vi "LC1_MS_Main.vi"(0 "MS_Network_Settings":T5, 1 "Analog Output":T1[](array[typedef]) {"value" format="%#_15f"}, 2 "Analog Input Indexes":u16[](array[numeric]), 3 "Digital Input Indexes":u16[](array[numeric]), 5 "MS_DNP3_Settings":T15={"Binary Out Mode"=6, "Binary In Variation"=0, "Analog Out Variation"=4, "Analog Out Mode"=6, "Analog In Variation"=6} {"Binary Out Mode" items=["SBO"=0, "Select"=3, "Operate"=4, "Direct"=5, "Direct No Ack"=6]; "Binary In Variation" items=["Default", "Packed Format", "With Flags"]; "Analog Out Variation" items=["32-bit"=1, "16-bit"=2, "Single-prec"=3, "Double-prec"=4]; "Analog Out Mode" items=["SBO"=0, "Select"=3, "Operate"=4, "Direct"=5, "Direct No Ack"=6]; "Analog In Variation" items=["Default", "32-bit with Flag", "16-bit with Flag", "32-bit without Flag", "16-bit without Flag", "Single-prec with Flag", "Double-prec with Flag"]}, 7 "MS_RESET":bool, 9 "MS_ENABLE":bool, 11 "Poll Enable":T13, 13 "Digital Output":T6[](array[typedef]) {"CROB value"."Control" items=["Nul"=0, "Pulse On"=1, "Pulse Off"=2, "Latch On"=3, "Latch Off"=4, "Close"=65, "Trip"=129]}, 14 "DNP3 Session Feedback":T4) -> (4 "Comm Status":T14, 6 "Analog Input":dbl[](array[numeric]), 8 "Digital Input":bool[](array[boolean]), 15 "DNP3 Session Output":T4)   [LabVIEW 2016, in "DNP3_Master_Station_MGCC.lvlib"]
uses:
  DNP3_Master_Station_MGCC.lvlib
  Tab_Master.ctl
  <vilib>/DNP3/DNP3_Master/Operation Mode.ctl
  <vilib>/DNP3/DNP3_Master/Poll Binary Input Variation.ctl
  <vilib>/DNP3/DNP3_Master/Analog Variation.ctl
  <vilib>/DNP3/DNP3_Master/Poll Analog Input Variation.ctl
  <vilib>/DNP3/DNP3_Master/Response Type.ctl
  <vilib>/DNP3/DNP3_Master/Analog Info.ctl
  <vilib>/DNP3/DNP3_Master/Start Stop.ctl
  <vilib>/DNP3/DNP3_Master/Crob With Index.ctl
  <vilib>/DNP3/DNP3_Common/crob.ctl
  <vilib>/DNP3/DNP3_Common/crob_ctrl.ctl
  <vilib>/Utility/error.llb/Error Cluster From Error Code.vi
  <vilib>/DNP3/DNP3_Master/Send CROB (Blocking).vi
  <vilib>/DNP3/DNP3_Master/Read Binary Input.vi
  <vilib>/DNP3/DNP3_Master/Send Poll Binary Input By StartStop (Blocking).vi
  <vilib>/DNP3/DNP3_Master/Send Analog Output Block (Blocking).vi
  <vilib>/DNP3/DNP3_Master/Read Analog Input.vi
  <vilib>/DNP3/DNP3_Master/Send Poll Analog Input By StartStop (Blocking).vi
  <vilib>/DNP3/DNP3_Master/Send Poll Analog Input By AllPoints (Blocking).vi
  <vilib>/ErrorRing/Error Ring.xnode
  <vilib>/DNP3/DNP3_Master.lvlib
  <resource>/objmgr/dnp3.rc
  <vilib>/DNP3/DNP3_Common.lvlib
panel:
  out "array w/ subset deleted":T1[](array[typedef]) {"value" format="%#_15f"}
  out "MS_Network_Settings_Initial 3":T5
  out "MS_Network_Settings_Initial 2":T5
  out "Ping status":T2=enum."Cancel"
  out "PollD":T3[](array[typedef])
  out "Array":T3[](array[typedef])
  out "PollA":T3[](array[typedef])
  out "Binary Out Mode":T9=6 items=["SBO"=0, "Select"=3, "Operate"=4, "Direct"=5, "Direct No Ack"=6]
  out "Binary In Variation":T10 items=["Default", "Packed Format", "With Flags"]
  out "Analog Out Variation":T11=4 items=["32-bit"=1, "16-bit"=2, "Single-prec"=3, "Double-prec"=4]
  out "Analog Out Mode":T9 items=["SBO"=0, "Select"=3, "Operate"=4, "Direct"=5, "Direct No Ack"=6]
  out "Analog In Variation":T12 items=["Default", "32-bit with Flag", "16-bit with Flag", "32-bit without Flag", "16-bit without Flag", "Single-prec with Flag", "Double-prec with Flag"]
  out "MS_TX_Status_Binary":T2
  out "MS_TX_Status_Analog":T2
  out "MS_RX_Status_Binary":T2
  out "MS_RX_Status_Analog":T2
  out "MS_Network_Settings_Initial":T5
  in  "En_Tx_Di":bool
  in  "En_Tx_An":bool
  in  "En_Rx_Di":bool
  in  "En_Rx_An":bool
  out "MS_RESET_IND":bool
  out "object flags":u8[](array[numeric]) format="%08b"
  in  "Channel Setting":T16
  in  "serial port":u16=1
  in  "baud rate (9600)":u32=9600
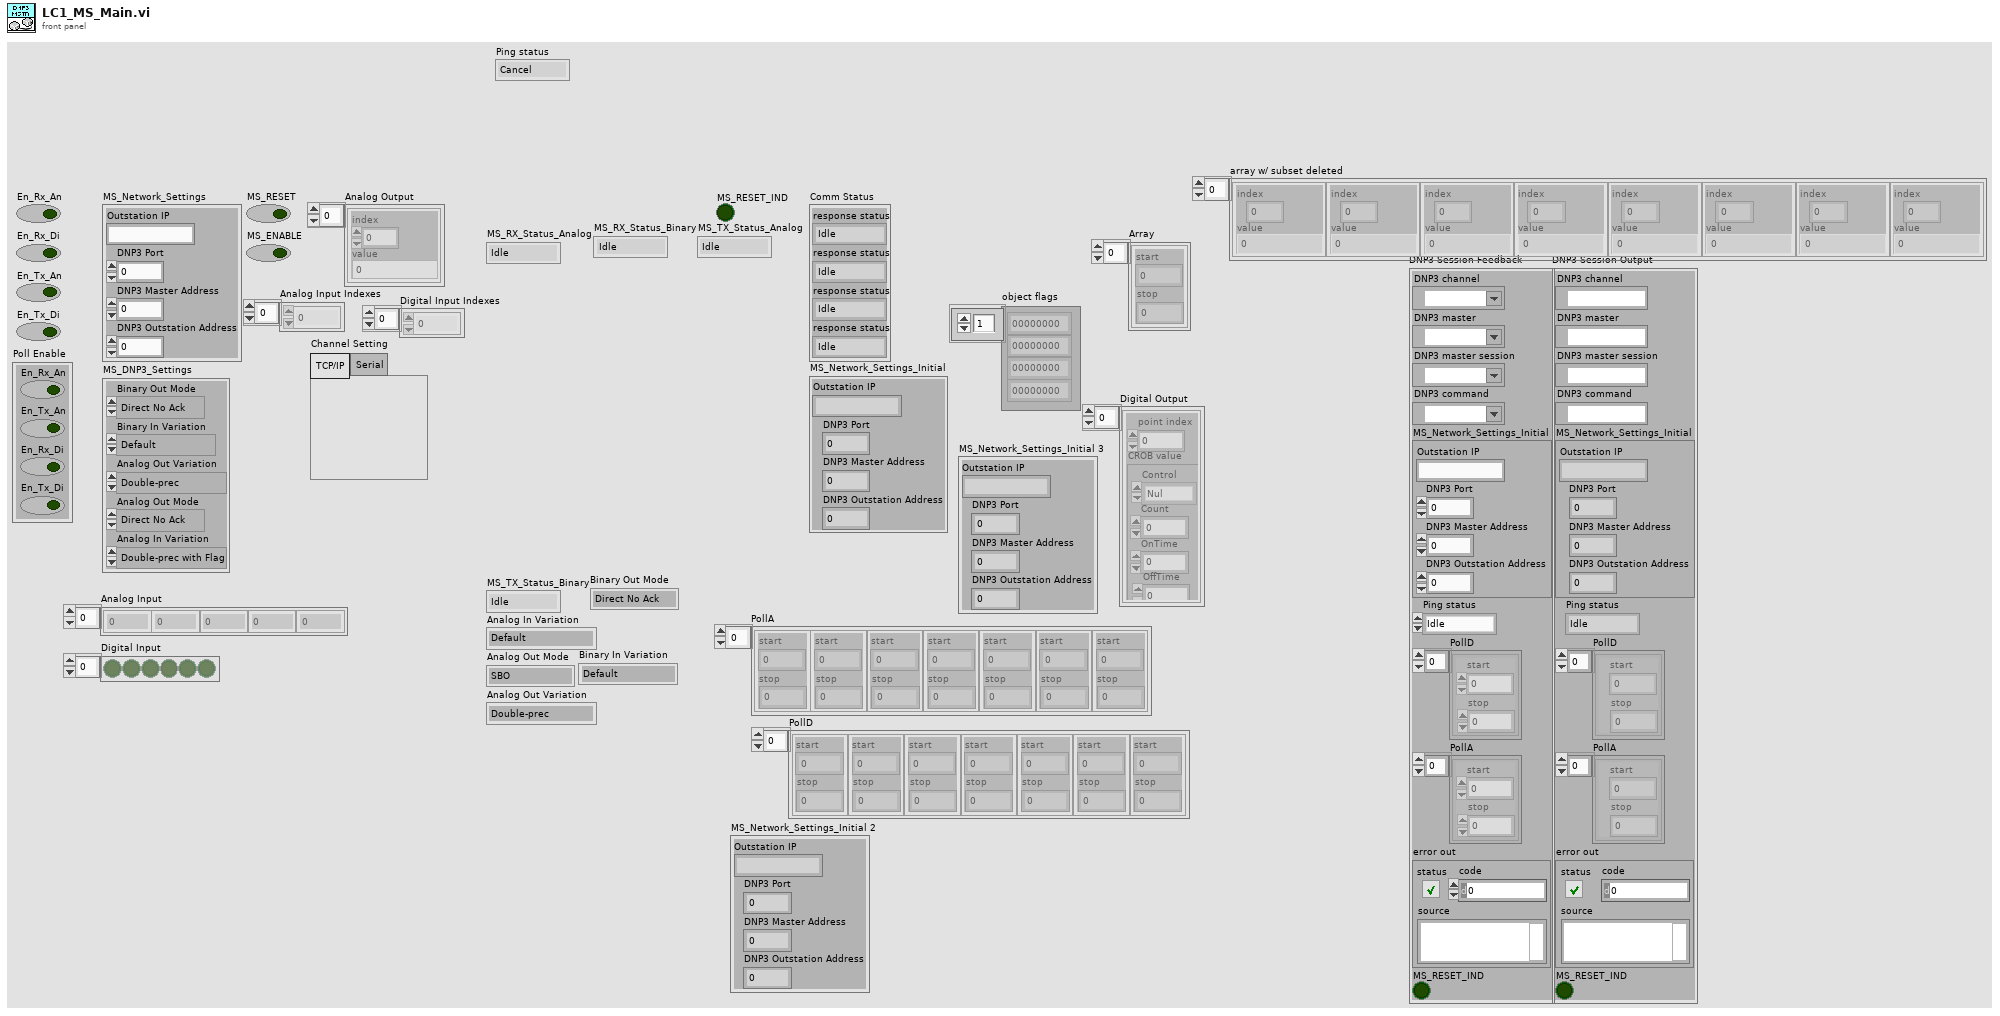
[diagram p1: front panel]
types:
  T1 = typedef "DNP3_Master.lvlib/Analog Info.ctl" = cluster{"index":u16, "value":dbl}
  T2 = typedef "DNP3_Master.lvlib/Response Type.ctl" = enum16{"Idle", "Buffering", "Pending", "Success", "Failure", "Mismatch", "Status Code", "IIN", "Timeout", "Cancel"}
  T3 = typedef "DNP3_Master.lvlib/Start Stop.ctl" = cluster{"start":u16, "stop":u16}
  T4 = cluster{"DNP3 channel":refnum<k21>, "DNP3 master":refnum<k21>, "DNP3 master session":refnum<k21>, "DNP3 command":refnum<k21>, "MS_Network_Settings_Initial":cluster{"Outstation IP":string, "DNP3 Port":u16, "DNP3 Master Address":u16, "DNP3 Outstation Address":u16}, "Ping status":T2, "PollD":T3[], "PollA":T3[], "error out":errorcluster, "MS_RESET_IND":bool}
  T5 = cluster{"Outstation IP":string, "DNP3 Port":u16, "DNP3 Master Address":u16, "DNP3 Outstation Address":u16}
  T6 = typedef "DNP3_Master.lvlib/Crob With Index.ctl" = cluster{"point index":u16, "CROB value":T7}
  T7 = typedef "DNP3_Common.lvlib/crob.ctl" = cluster{"OnTime":u32, "Count":u8, "OffTime":u32, "Control":T8}
  T8 = typedef "DNP3_Common.lvlib/crob_ctrl.ctl" = u8
  T9 = typedef "DNP3_Master.lvlib/Operation Mode.ctl" = u8
  T10 = typedef "DNP3_Master.lvlib/Poll Binary Input Variation.ctl" = u8
  T11 = typedef "DNP3_Master.lvlib/Analog Variation.ctl" = u8
  T12 = typedef "DNP3_Master.lvlib/Poll Analog Input Variation.ctl" = u8
  T13 = cluster{"En_Rx_An":bool, "En_Tx_An":bool, "En_Rx_Di":bool, "En_Tx_Di":bool}
  T14 = cluster{"response status":T2, "response status":T2, "response status":T2, "response status":T2}
  T15 = cluster{"Binary Out Mode":T9, "Binary In Variation":T10, "Analog Out Variation":T11, "Analog Out Mode":T9, "Analog In Variation":T12}
  T16 = typedef "Tab_Master.ctl" = enum32{"TCP/IP", "Serial"}
  T17 = cluster{"Analog RX":T2, "Analog RX":T2, "Analog RX":T2, "Analog RX":T2}
  T18 = cluster{"DNP3 Master Address":u16, "DNP3 Outstation Address":u16}
  T19 = cluster{"x = y?":bool, "Outstation IP":string, "DNP3 Port":u16, "serial port":u16, "baud rate (9600)":u32}
  T20 = cluster{"MS_RX_Status_Analog":T2, "MS_TX_Status_Analog":T2, "MS_RX_Status_Binary":T2, "MS_TX_Status_Binary":T2}
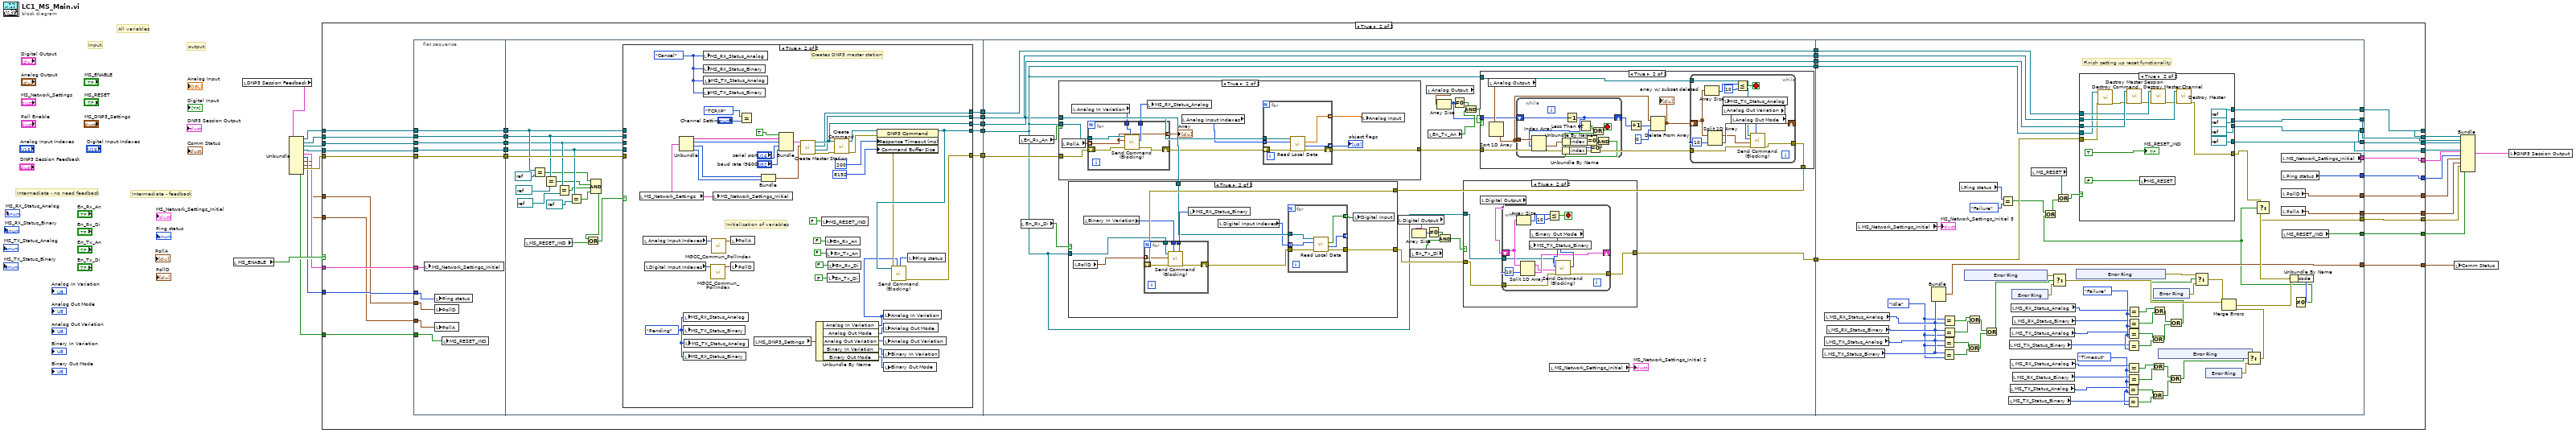
[diagram p0: block diagram]
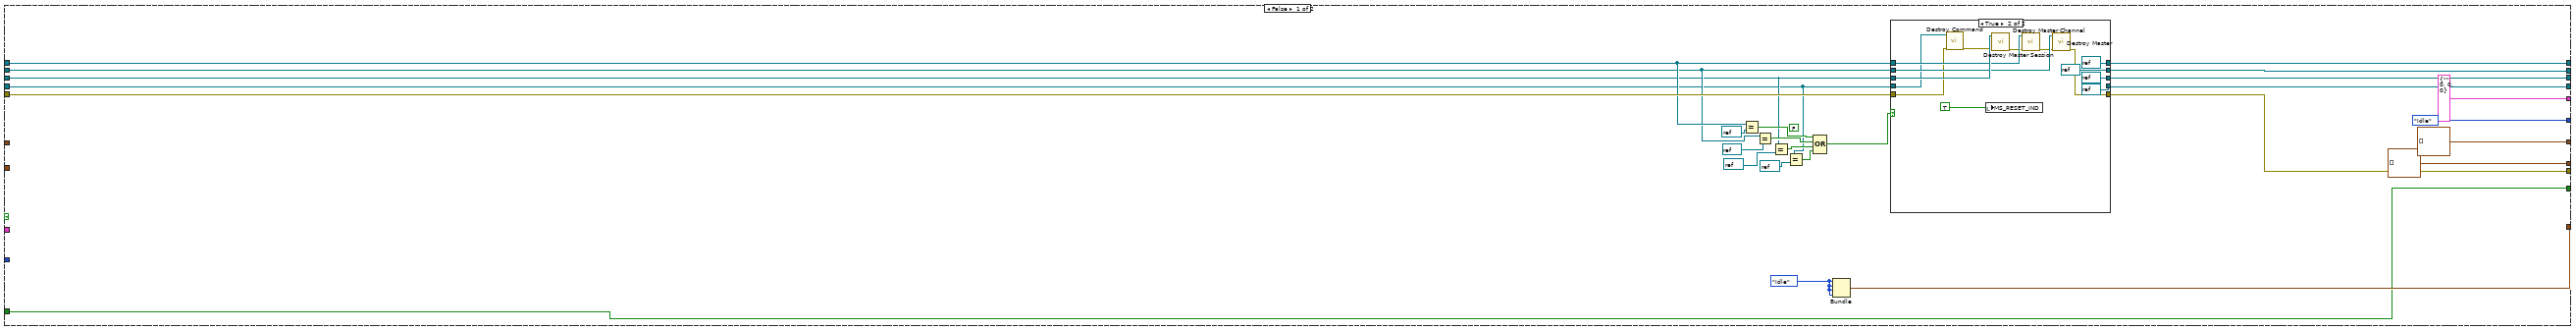
[diagram p2: hidden frame]
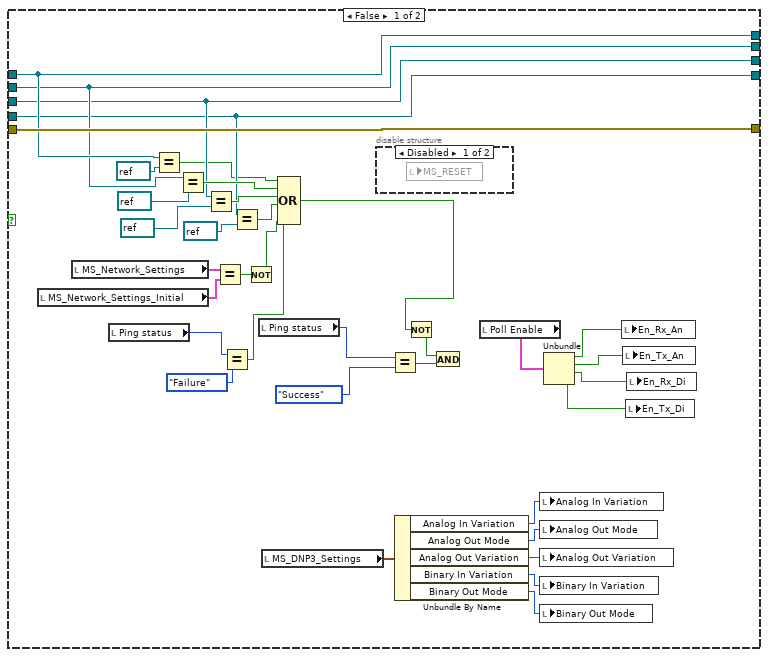
[diagram p4: hidden frame]
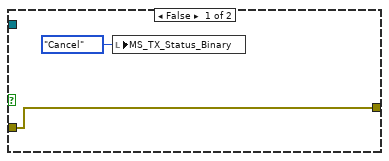
[diagram p6: hidden frame]
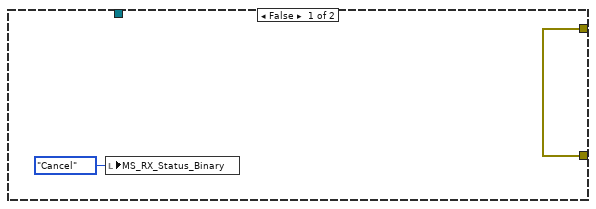
[diagram p7: hidden frame]
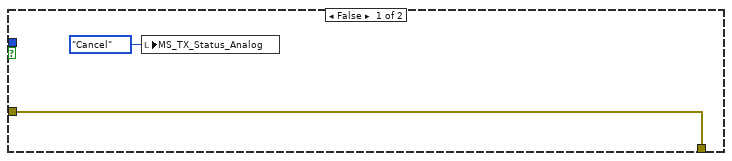
[diagram p8: hidden frame]
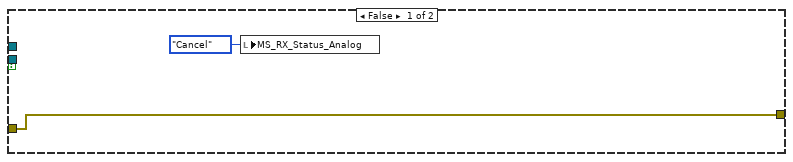
[diagram p9: hidden frame]
diagram:
  # "Intermediate - feedback"
  # "Intermediate - no need feedback"
  # "output"
  # "Input"
  # "All variables"
  n1 = local read "MS_ENABLE"() -> (w17:bool)
  n2 = local read "DNP3 Session Feedback"() -> (w9:T4)
  n3 = Unbundle(w9) -> ("DNP3 channel"=w24:refnum<k21>, "DNP3 master"=w23:refnum<k21>, "DNP3 master session"=w21:refnum<k21>, "DNP3 command"=w22:refnum<k21>, "MS_Network_Settings_Initial"=w7:T5, "Ping status"=w6:T2, "PollD"=w5:T3[], "PollA"=w4:T3[], "error out"=w8:errorcluster, "MS_RESET_IND"=w1:bool)
  n4 = case shown="True" w17 {
    tunnel: w23 -> [w32 w105]
    tunnel: w21 -> [w31 w104]
    tunnel: w22 -> [w30 w103]
    tunnel: [w45 w86] -> w19
    tunnel: w8 -> [w48 w102]
    tunnel: [w47 w89] -> w10
    tunnel: [w44 w85] -> w18
    tunnel: [w43 w88] -> w15
    tunnel: [w46 w87] -> w20
    tunnel: w24 -> [w33 w101]
    tunnel: [w50 w90] -> w16
    tunnel: [T5 {"Outstation IP"="", "DNP3 Port"=0, "DNP3 Master Address"=0, "DNP3 Outstation Address"=0} ("MS_Network_Settings_Initial") w75] -> w14
    tunnel: [Response_Type."Idle" ("Ping status") w74] -> w13
    tunnel: [T3[] [] ("PollD") w73] -> w12
    tunnel: [T3[] [] ("PollA") w72] -> w11
    tunnel: w7 -> [_ w84]
    tunnel: w6 -> [_ w83]
    tunnel: w5 -> [_ w82]
    tunnel: w4 -> [_ w81]
    tunnel: [w25 w71] -> w3
    tunnel: w1 -> [w25 w70]
    frame False {
      (unwired) FALSE ("value")
      w49 = Response_Type."Idle" ("Analog RX")
      n5 = Equal?(x=w33, y=refnum<k21> refnum ("DNP3 channel")) -> (x = y?=w35:bool)
      n6 = Equal?(x=w32, y=refnum<k21> refnum) -> (x = y?=w37:bool)
      n7 = Equal?(x=w31, y=refnum<k21> refnum) -> (x = y?=w38:bool)
      n8 = Equal?(x=w30, y=refnum<k21> refnum) -> (x = y?=w39:bool)
      n9 = Compound Arithmetic op=OR(w35, w37, w38, w39) -> (w34:bool)
      n10 = Bundle("Analog RX"=w49, "Analog RX"=w49, "Analog RX"=w49, "Analog RX"=w49) -> (w50:T17)  [unwired: 1 in]
      n11 = case shown="True" w34 {
        tunnel: w31 -> [w52 w69]
        tunnel: w48 -> [w55 w61]
        tunnel: w33 -> [w54 w68]
        tunnel: w32 -> [w53 w67]
        tunnel: [w55 w66] -> w47
        tunnel: w30 -> [w51 w62]
        tunnel: [w54 refnum<k21> refnum ("DNP3 channel")] -> w46
        tunnel: [w53 refnum<k21> refnum ("DNP3 master")] -> w45
        tunnel: [w52 refnum<k21> refnum ("DNP3 master session")] -> w44
        tunnel: [w51 refnum<k21> refnum ("DNP3 command")] -> w43
        frame False {
        }
        frame True {
          n12 = call <vilib>:"Destroy Command.vi"("error in (no error)"=w61, "DNP3 command in"=w62) -> ("error out"=w60:errorcluster)  [unwired: 8 in, 1 out]
          n13 = local write "MS_RESET_IND"(TRUE ("MS_Comm_Reset_Succesful")) -> ()
          n14 = call <vilib>:"Destroy Master Session.vi"("error in (no error)"=w60, "DNP3 master session in"=w69) -> ("error out"=w65:errorcluster)  [unwired: 8 in, 1 out]
          n15 = call <vilib>:"Destroy Master Channel.vi"("error in (no error)"=w65, "DNP3 channel in"=w68) -> ("error out"=w64:errorcluster)  [unwired: 8 in, 1 out]
          n16 = call <vilib>:"Destroy Master.vi"("error in (no error)"=w64, "DNP3 master"=w67) -> ("error out"=w66:errorcluster)  [unwired: 9 in]
        }
      }
    }
    frame True {
      n17 = flat-sequence {
        tunnel: w81 -> [w107]
        tunnel: w82 -> [w108]
        tunnel: w83 -> [w109]
        tunnel: w84 -> [w110]
        tunnel: w101 -> [w111]
        tunnel: w102 -> [w112]
        tunnel: w103 -> [w113]
        tunnel: w104 -> [w114]
        tunnel: w105 -> [w115]
        tunnel: [w115] -> w80
        tunnel: [w114] -> w79
        tunnel: [w113] -> w78
        tunnel: [w112] -> w77
        tunnel: [w111] -> w76
        tunnel: w70 -> [w106]
        tunnel: [w136] -> w100
        tunnel: [w135] -> w99
        tunnel: [w133] -> w98
        tunnel: [w132] -> w97
        tunnel: [w131] -> w96
        tunnel: w80 -> [w126]
        tunnel: w79 -> [w125]
        tunnel: w78 -> [w124]
        tunnel: w77 -> [w134]
        tunnel: w76 -> [w129]
        tunnel: w100 -> [w221]
        tunnel: w99 -> [w219]
        tunnel: w98 -> [w217]
        tunnel: w97 -> [w220]
        tunnel: w96 -> [w218]
        tunnel: [w220] -> w95
        tunnel: [w219] -> w94
        tunnel: [w218] -> w93
        tunnel: [w217] -> w92
        tunnel: [w216] -> w91
        tunnel: w95 -> [w411]
        tunnel: w94 -> [w410]
        tunnel: w93 -> [w409]
        tunnel: w92 -> [w408]
        tunnel: w91 -> [w407]
        tunnel: [w360] -> w90
        tunnel: [w359] -> w89
        tunnel: [w358] -> w88
        tunnel: [w356] -> w87
        tunnel: [w355] -> w86
        tunnel: [w354] -> w85
        tunnel: [w351] -> w75
        tunnel: [w350] -> w74
        tunnel: [w349] -> w73
        tunnel: [w348] -> w72
        tunnel: [w347] -> w71
        frame #0 {
          n18 = local write "MS_Network_Settings_Initial"(w110) -> ()
          n19 = local write "Ping status"(w109) -> ()
          n20 = local write "PollD"(w108) -> ()
          n21 = local write "PollA"(w107) -> ()
          n22 = local write "MS_RESET_IND"(w106) -> ()
        }
        frame #1 {
          n23 = local read "MS_RESET_IND"() -> (w130:bool)
          n24 = Equal?(x=w129, y=refnum<k21> refnum ("DNP3 channel")) -> (x = y?=w123:bool)
          n25 = Equal?(x=w126, y=refnum<k21> refnum) -> (x = y?=w122:bool)
          n26 = Equal?(x=w125, y=refnum<k21> refnum) -> (x = y?=w121:bool)
          n27 = Equal?(x=w124, y=refnum<k21> refnum) -> (x = y?=w120:bool)
          n28 = Compound Arithmetic op=AND(w123, w122, w121, w120) -> (w116:bool)
          n29 = Or(x=w116, y=w130) -> (x .or. y?=w127:bool)
          n30 = case shown="True" w127 {
            tunnel: [w172 w192] -> w136
            tunnel: [w153 w194] -> w131
            tunnel: [w154 w208] -> w133
            tunnel: w126 -> [w155 _]
            tunnel: w125 -> [w154 _]
            tunnel: w124 -> [w153 _]
            tunnel: [w155 w195] -> w135
            tunnel: w134 -> [w172 _]
            tunnel: [w156 w196] -> w132
            tunnel: w129 -> [w156 _]
            frame False {
              n31 = local read "MS_Network_Settings_Initial"() -> (w147:T5)
              n32 = local read "MS_Network_Settings"() -> (w148:T5)
              n33 = local read "Ping status"() -> (w144:T2)
              n34 = Equal?(x=w156, y=refnum<k21> refnum ("DNP3 channel")) -> (x = y?=w152:bool)
              n35 = Equal?(x=w155, y=refnum<k21> refnum) -> (x = y?=w158:bool)
              n36 = Equal?(x=w154, y=refnum<k21> refnum) -> (x = y?=w159:bool)
              n37 = Equal?(x=w148, y=w147) -> (x = y?=w149:bool)
              n38 = Equal?(x=w144, y=Response_Type."Failure" ("Ping status")) -> (x = y?=w142:bool)
              n39 = Equal?(x=w153, y=refnum<k21> refnum) -> (x = y?=w160:bool)
              n40 = Not(x=w149) -> (.not. x?=w146:bool)
              n41 = local read "Ping status"() -> (w171:T2)
              n42 = local read "MS_DNP3_Settings"() -> (w169:T15)
              n43 = Compound Arithmetic op=OR(w152, w158, w159, w160, w146, w142) -> (w145:bool)
              n44 = disable-structure shown="Disabled" {
                frame Disabled {
                  n45 = local read "MS_RESET"() -> ()  [unwired: 1 in]
                }
                frame Enabled {
                }
              }
              n46 = Equal?(x=w171, y=Response_Type."Success" ("Ping status")) -> (x = y?=w151:bool)
              n47 = Unbundle By Name(w169) -> ("Analog In Variation"=w168:T12, "Analog Out Mode"=w167:T9, "Analog Out Variation"=w166:T11, "Binary In Variation"=w165:T10, "Binary Out Mode"=w164:T9)
              n48 = Not(x=w145) -> (.not. x?=w150:bool)
              n49 = And(x=w150, y=w151) -> ()  [unwired: 1 out]
              n50 = local read "Poll Enable"() -> (w137:T13)
              n51 = local write "Analog In Variation"(w168) -> ()
              n52 = local write "Analog Out Mode"(w167) -> ()
              n53 = local write "Analog Out Variation"(w166) -> ()
              n54 = local write "Binary In Variation"(w165) -> ()
              n55 = local write "Binary Out Mode"(w164) -> ()
              n56 = Unbundle(w137) -> ("En_Rx_An"=w138:bool, "En_Tx_An"=w139:bool, "En_Rx_Di"=w140:bool, "En_Tx_Di"=w141:bool)
              n57 = local write "En_Rx_An"(w138) -> ()
              n58 = local write "En_Tx_An"(w139) -> ()
              n59 = local write "En_Tx_Di"(w141) -> ()
              n60 = local write "En_Rx_Di"(w140) -> ()
            }
            frame True {
              w182 = Response_Type."Pending" ("LC1_MS_RX_Status_Binary")
              w197 = Response_Type."Cancel" ("LC1_MS_RX_Status_Binary")
              # "Initialization of variables"
              # "Creates DNP3 master station"
              n61 = local read "MS_Network_Settings"() -> (w180:T5)
              n62 = local read "Analog Input Indexes"() -> (w187:u16[])
              n63 = local read "Digital Input Indexes"() -> (w186:u16[])
              n64 = Unbundle(w180) -> ("Outstation IP"=w207:string, "DNP3 Port"=w206:u16, "DNP3 Master Address"=w205:u16, "DNP3 Outstation Address"=w204:u16)
              n65 = local write "MS_RX_Status_Analog"(w182) -> ()
              n66 = local write "MS_TX_Status_Binary"(w182) -> ()
              n67 = local write "MS_RX_Status_Binary"(w182) -> ()
              n68 = local write "MS_TX_Status_Analog"(w182) -> ()
              n69 = local write "MS_RX_Status_Analog"(w197) -> ()
              n70 = local write "MS_RX_Status_Binary"(w197) -> ()
              n71 = local write "MS_TX_Status_Binary"(w197) -> ()
              n72 = local write "MS_TX_Status_Analog"(w197) -> ()
              n73 = call "MGCC_Commun_PollIndex.vi"("Analog Input Indexes"=w186) -> ("Poll"=w183:T3[])  [unwired: 10 in]
              n74 = call "MGCC_Commun_PollIndex.vi"("Analog Input Indexes"=w187) -> ("Poll"=w184:T3[])  [unwired: 10 in]
              n75 = local write "MS_Network_Settings_Initial"(w180) -> ()
              n76 = local write "PollD"(w183) -> ()
              n77 = local write "PollA"(w184) -> ()
              n78 = Equal?(x=Tab_Master."TCP/IP" ("Channel Setting"), y="Channel Setting") -> ()  [unwired: 1 out]
              n79 = local read "MS_DNP3_Settings"() -> (w179:T15)
              n80 = Bundle("DNP3 Master Address"=w205, "DNP3 Outstation Address"=w204) -> (w202:T18)  [unwired: 1 in]
              n81 = Bundle("x = y?"=TRUE, "Outstation IP"=w207, "DNP3 Port"=w206, "serial port"="serial port", "baud rate (9600)"="baud rate (9600)") -> (w203:T19)  [unwired: 1 in]
              n82 = call "Create Master Station.vi"("Session Cluster"=w202, "Channel Cluster"=w203) -> ("error out"=w210:errorcluster, "DNP3 master"=w195:refnum<k21>, "DNP3 channel"=w196:refnum<k21>, "DNP3 master session"=w208:refnum<k21>)  [unwired: 3 in]
              n83 = Unbundle By Name(w179) -> ("Analog In Variation"=w174:T12, "Analog Out Mode"=w178:T9, "Analog Out Variation"=w177:T11, "Binary In Variation"=w176:T10, "Binary Out Mode"=w175:T9)
              n84 = local write "MS_RESET_IND"(FALSE ("MS_Comm_Reset_Ind")) -> ()
              n85 = local write "En_Rx_An"(FALSE ("En_Rx_An")) -> ()
              n86 = local write "En_Tx_An"(FALSE ("En_Tx_An")) -> ()
              n87 = local write "En_Tx_Di"(FALSE ("En_Tx_Di")) -> ()
              n88 = local write "En_Rx_Di"(FALSE ("En_Rx_Di")) -> ()
              n89 = call <vilib>:"Create Command.vi"("error in (no error)"=w210, "DNP3 master session"=w208) -> ("error out"=w200:errorcluster, "DNP3 command"=w201:refnum<k21>)  [unwired: 8 in]
              n90 = property class="DNP3 Command"(reference=w201, error in=w200, "Response Timeout (ms)"=u32 200 ("Misc:Response Timeout (ms)"), "Command Buffer Size"=u32 8192 ("Misc:Command Buffer Size")) -> (reference out=w194:refnum<k21>, error out=w193:errorcluster)
              n91 = local write "Analog In Variation"(w174) -> ()
              n92 = local write "Analog Out Mode"(w178) -> ()
              n93 = local write "Analog Out Variation"(w177) -> ()
              n94 = local write "Binary In Variation"(w176) -> ()
              n95 = local write "Binary Out Mode"(w175) -> ()
              n96 = call-poly <vilib>:"Send Command (Blocking).vi"("variation (Default)"=w174, "error in (no error)"=w193, "DNP3 command in"=w194) -> ("error out"=w192:errorcluster, "response status"=w181:T2)  [unwired: 6 in, 1 out]
              n97 = local write "Ping status"(w181) -> ()
            }
          }
        }
        frame #2 {
          n98 = local read "En_Rx_An"() -> (w232:bool)
          n99 = local read "En_Rx_Di"() -> (w233:bool)
          n100 = case shown="True" w232 {
            tunnel: w221 -> [w316 w328]
            tunnel: w217 -> [_ w322]
            tunnel: w218 -> [_ w327]
            tunnel: [w316 w325] -> w222
            frame False {
              n101 = local write "MS_RX_Status_Analog"(Response_Type."Cancel" ("MS_RX_Status_Analog")) -> ()
            }
            frame True {
              n102 = local read "PollA"() -> (w320:T3[])
              n103 = local read "Analog In Variation"() -> (w323:T12)
              n104 = for {
                tunnel: w327 -> [w333]
                tunnel: [w332] -> w324
                tunnel: w323 -> [w331]
                shift-right: [w330] -> w321
                shift-left: w328 -> [w334]
                tunnel: w320 -> [w329] mode=indexing
                tunnel: [w329] -> w318 mode=indexing
                n105 = call-poly <vilib>:"Send Command (Blocking).vi"("variation (Default)"=w331, "error in (no error)"=w334, "range"=w329, "DNP3 command in"=w333) -> ("error out"=w330:errorcluster, "response status"=w332:T2)  [unwired: 5 in, 1 out]
              }
              "Array" <- w318
              n106 = local write "MS_RX_Status_Analog"(w324) -> ()
              n107 = local read "Analog Input Indexes"() -> (w319:u16[])
              n108 = for {
                tunnel: [w338] -> w317 mode=indexing
                tunnel: [w337] -> w326 mode=indexing
                tunnel: w322 -> [w336]
                tunnel: w319 -> [w335] mode=indexing
                shift-right: [w339] -> w325
                shift-left: w321 -> [w340]
                n109 = call-poly <vilib>:"Read Local Data.vi"("error in (no error)"=w340, "point index"=w335, "DNP3 master session in"=w336) -> ("error out"=w339:errorcluster, "object flags"=w337:u8, "value"=w338:dbl)  [unwired: 5 in, 1 out]
              }
              "object flags" <- w326
              n110 = local write "Analog Input"(w317) -> ()
            }
          }
          n111 = local read "Digital Output"() -> (w231:T6[])
          n112 = local read "En_Tx_Di"() -> (w235:bool)
          n113 = Array Size(array=w231) -> (size(s)=w228:i32)
          n114 = local read "Analog Output"() -> (w227:T1[])
          n115 = Not Equal To 0?(x=w228) -> (x != 0?=w229:bool)
          n116 = local read "En_Tx_An"() -> (w234:bool)
          n117 = Array Size(array=w227) -> (size(s)=w214:i32)
          n118 = And(x=w229, y=w235) -> (x .and. y?=w230:bool)
          n119 = Not Equal To 0?(x=w214) -> (x != 0?=w226:bool)
          n120 = And(x=w226, y=w234) -> (x .and. y?=w225:bool)
          n121 = case shown="True" w225 {
            tunnel: w218 -> [_ w288]
            tunnel: w222 -> [w279 w289]
            tunnel: [w279 w287] -> w223
            tunnel: w214 -> [_ w283]
            frame False {
              n122 = local write "MS_TX_Status_Analog"(Response_Type."Cancel" ("MS_TX_Status_Analog")) -> ()
            }
            frame True {
              n123 = local read "Analog Output"() -> (w284:T1[])
              n124 = Sort 1D Array(array=w284) -> (sorted array=w280:T1[])
              n125 = while {
                shift-right: [w290] -> w281
                shift-left: w283 -> [w297]
                tunnel: w280 -> [w295]
                stop <- w301 stop-if-true
                n126 = Decrement(x=w297) -> (x-1=w290:i32)
                n127 = Index Array(array=w295, index #1=w290) -> (element #1=w292:T1, element #2=w291:T1)  [unwired: 1 in]
                n128 = Unbundle By Name(w291) -> ("index"=w294:u16)
                n129 = Unbundle By Name(w292) -> ("index"=w293:u16)
                n130 = Less Than 0?(x=w290) -> (x < 0?=w296:bool)
                n131 = Equal To 0?(x=w293) -> (x = 0?=w300:bool)
                n132 = Equal To 0?(x=w294) -> (x = 0?=w299:bool)
                n133 = And(x=w300, y=w299) -> (x .and. y?=w298:bool)
                n134 = Or(x=w296, y=w298) -> (x .or. y?=w301:bool)
              }
              n135 = Increment(x=w281) -> (x+1=w282:i32)
              n136 = Delete From Array(array=w280, length=w282, index=0) -> (array with subset deleted=w286:T1[])  [unwired: 1 out]
              "array w/ subset deleted" <- w286
              n137 = while {
                shift-right: [w306] -> _
                shift-left: w286 -> [w310]
                tunnel: [w305] -> w287
                tunnel: w288 -> [w304]
                tunnel: w289 -> [w302]
                stop <- w311 stop-if-true
                n138 = Array Size(array=w310) -> (size(s)=w313:i32)
                n139 = Split 1D Array(array=w310, index=10) -> (first subarray=w303:T1[], second subarray=w306:T1[])
                n140 = local read "Analog Out Variation"() -> (w307:T11)
                n141 = local read "Analog Out Mode"() -> (w308:T9)
                n142 = Less Or Equal?(x=w313, y=10) -> (x <= y?=w311:bool)
                n143 = call-poly <vilib>:"Send Command (Blocking).vi"("variation"=w307, "error in (no error)"=w302, "values"=w303, "mode"=w308, "DNP3 command in"=w304) -> ("error out"=w305:errorcluster, "response status"=w309:T2)  [unwired: 4 in, 1 out]
                n144 = local write "MS_TX_Status_Analog"(w309) -> ()
              }
            }
          }
          n145 = case shown="True" w233 {
            tunnel: w217 -> [_ w260]
            tunnel: w218 -> [_ w257]
            tunnel: w223 -> [w255 w265]
            tunnel: [w255 w264] -> w224
            frame False {
              n146 = local write "MS_RX_Status_Binary"(Response_Type."Cancel" ("MS_RX_Status_Binary")) -> ()
            }
            frame True {
              n147 = local read "PollD"() -> (w258:T3[])
              n148 = local read "Binary In Variation"() -> (w261:T10)
              n149 = for {
                tunnel: [w269] -> w262
                tunnel: w261 -> [w268]
                shift-right: [w270] -> w263
                shift-left: w265 -> [w271]
                tunnel: w258 -> [w267] mode=indexing
                tunnel: w257 -> [w266]
                n150 = call-poly <vilib>:"Send Command (Blocking).vi"("variation (Default)"=w268, "error in (no error)"=w271, "range"=w267, "DNP3 command in"=w266) -> ("error out"=w270:errorcluster, "response status"=w269:T2)  [unwired: 5 in, 1 out]
              }
              n151 = local write "MS_RX_Status_Binary"(w262) -> ()
              n152 = local read "Digital Input Indexes"() -> (w259:u16[])
              n153 = for {
                tunnel: [w277] -> w264
                tunnel: [w276] -> _ mode=indexing
                tunnel: [w275] -> w256 mode=indexing
                tunnel: w260 -> [w274]
                tunnel: w259 -> [w273] mode=indexing
                tunnel: w263 -> [w272]
                n154 = call-poly <vilib>:"Read Local Data.vi"("error in (no error)"=w272, "point index"=w273, "DNP3 master session in"=w274) -> ("error out"=w277:errorcluster, "object flags"=w276:u8, "value"=w275:bool)  [unwired: 5 in, 1 out]
              }
              n155 = local write "Digital Input"(w256) -> ()
            }
          }
          n156 = case shown="True" w230 {
            tunnel: [w237 w240] -> w216
            tunnel: w224 -> [w237 w241]
            tunnel: w218 -> [_ w239]
            frame False {
              n157 = local write "MS_TX_Status_Binary"(Response_Type."Cancel" ("MS_TX_Status_Binary")) -> ()
            }
            frame True {
              n158 = local read "Digital Output"() -> (w238:T6[])
              n159 = while {
                shift-right: [w246] -> _
                shift-left: w238 -> [w249]
                tunnel: w241 -> [w245]
                tunnel: [w244] -> w240
                tunnel: w239 -> [w242]
                stop <- w250 stop-if-true
                n160 = Array Size(array=w249) -> (size(s)=w252:i32)
                n161 = Split 1D Array(array=w249, index=10) -> (first subarray=w243:T6[], second subarray=w246:T6[])
                n162 = local read "Binary Out Mode"() -> (w248:T9)
                n163 = Less Or Equal?(x=w252, y=10) -> (x <= y?=w250:bool)
                n164 = call-poly <vilib>:"Send Command (Blocking).vi"("error in (no error)"=w245, "CROB values"=w243, "mode"=w248, "DNP3 command in"=w242) -> ("error out"=w244:errorcluster, "response status"=w247:T2)  [unwired: 5 in, 1 out]
                n165 = local write "MS_TX_Status_Binary"(w247) -> ()
              }
            }
          }
          n166 = local read "MS_Network_Settings_Initial"() -> (→"MS_Network_Settings_Initial 2":T5)
        }
        frame #3 {
          w386 = Response_Type."Timeout" ("Analog RX")
          w385 = Response_Type."Failure" ("Analog RX")
          w361 = Response_Type."Idle" ("Analog RX")
          # "Finish setting up reset functionality"
          n167 = local read "MS_TX_Status_Binary"() -> (w371:T2)
          n168 = local read "MS_TX_Status_Analog"() -> (w370:T2)
          n169 = local read "MS_RX_Status_Analog"() -> (w368:T2)
          n170 = local read "MS_RX_Status_Binary"() -> (w369:T2)
          n171 = local read "MS_Network_Settings_Initial"() -> (→"MS_Network_Settings_Initial 3":T5)
          n172 = Bundle("MS_RX_Status_Analog"=w368, "MS_TX_Status_Analog"=w370, "MS_RX_Status_Binary"=w369, "MS_TX_Status_Binary"=w371) -> (w360:T20)  [unwired: 1 in]
          n173 = Equal?(x=w370, y=w361) -> (x = y?=w366:bool)
          n174 = Equal?(x=w371, y=w361) -> (x = y?=w365:bool)
          n175 = Equal?(x=w361, y=w368) -> (x = y?=w364:bool)
          n176 = Equal?(x=w369, y=w361) -> (x = y?=w367:bool)
          n177 = local read "Ping status"() -> (w343:T2)
          n178 = xnode "Error Ring"() -> ("error out"=w379:errorcluster)
          n179 = Or(x=w366, y=w365) -> (x .or. y?=w363:bool)
          n180 = Or(x=w364, y=w367) -> (x .or. y?=w362:bool)
          n181 = Or(x=w362, y=w363) -> (x .or. y?=w380:bool)
          n182 = Equal?(x=w343, y=Response_Type."Failure" ("Analog RX")) -> (x = y?=w341:bool)
          n183 = local read "MS_TX_Status_Binary"() -> (w387:T2)
          n184 = local read "MS_TX_Status_Binary"() -> (w384:T2)
          n185 = local read "MS_TX_Status_Analog"() -> (w394:T2)
          n186 = local read "MS_TX_Status_Analog"() -> (w372:T2)
          n187 = local read "MS_RX_Status_Analog"() -> (w389:T2)
          n188 = local read "MS_RX_Status_Analog"() -> (w382:T2)
          n189 = xnode "Error Ring"() -> ("error out"=w378:errorcluster)
          n190 = local read "MS_RX_Status_Binary"() -> (w388:T2)
          n191 = local read "MS_RX_Status_Binary"() -> (w383:T2)
          n192 = local read "MS_RESET"() -> (w412:bool)
          n193 = Select(t=w379, s=w380, f=w378) -> (s? t:f=w402:errorcluster)
          n194 = xnode "Error Ring"() -> ("error out"=w396:errorcluster)
          n195 = Equal?(x=w394, y=w386) -> (x = y?=w392:bool)
          n196 = Equal?(x=w387, y=w386) -> (x = y?=w391:bool)
          n197 = Equal?(x=w372, y=w385) -> (x = y?=w374:bool)
          n198 = Equal?(x=w384, y=w385) -> (x = y?=w375:bool)
          n199 = Equal?(x=w389, y=w386) -> (x = y?=w390:bool)
          n200 = Equal?(x=w388, y=w386) -> (x = y?=w393:bool)
          n201 = Equal?(x=w382, y=w385) -> (x = y?=w381:bool)
          n202 = Equal?(x=w383, y=w385) -> (x = y?=w373:bool)
          n203 = Or(x=w392, y=w391) -> (x .or. y?=w353:bool)
          n204 = Or(x=w374, y=w375) -> (x .or. y?=w376:bool)
          n205 = Or(x=w390, y=w393) -> (x .or. y?=w395:bool)
          n206 = Or(x=w381, y=w373) -> (x .or. y?=w377:bool)
          n207 = xnode "Error Ring"() -> ("error out"=w397:errorcluster)
          n208 = xnode "Error Ring"() -> ("error out"=w399:errorcluster)
          n209 = Or(x=w395, y=w353) -> (x .or. y?=w401:bool)
          n210 = Or(x=w377, y=w376) -> (x .or. y?=w400:bool)
          n211 = Select(t=w396, s=w400, f=w397) -> (s? t:f=w403:errorcluster)
          n212 = xnode "Error Ring"() -> ("error out"=w398:errorcluster)
          n213 = Select(t=w399, s=w401, f=w398) -> (s? t:f=w404:errorcluster)
          n214 = Merge Errors(w402, w403, w404) -> (w405:errorcluster)
          n215 = local read "MS_Network_Settings_Initial"() -> (w351:T5)
          n216 = local read "Ping status"() -> (w350:T2)
          n217 = local read "PollD"() -> (w349:T3[])
          n218 = local read "PollA"() -> (w348:T3[])
          n219 = local read "MS_RESET_IND"() -> (w347:bool)
          n220 = Unbundle By Name(w405) -> ("code"=w406:i32)
          n221 = Not Equal To 0?(x=w406) -> (x != 0?=w345:bool)
          n222 = Or(x=w341, y=w345) -> (x .or. y?=w344:bool)
          n223 = Or(x=w412, y=w344) -> (x .or. y?=w346:bool)
          n224 = case shown="True" w346 {
            tunnel: w410 -> [w435 w451]
            tunnel: [w435 refnum<k21> refnum ("DNP3 master")] -> w355
            tunnel: w407 -> [w434 w441]
            tunnel: [w434 w448] -> w357
            tunnel: [w433 refnum<k21> refnum ("DNP3 master session")] -> w354
            tunnel: w408 -> [w433 w453]
            tunnel: [w432 refnum<k21> refnum ("DNP3 command")] -> w358
            tunnel: w409 -> [w432 w442]
            tunnel: w411 -> [w431 w452]
            tunnel: [w431 refnum<k21> refnum ("DNP3 channel")] -> w356
            frame False {
            }
            frame True {
              n225 = call <vilib>:"Destroy Command.vi"("error in (no error)"=w441, "DNP3 command in"=w442) -> ("error out"=w440:errorcluster)  [unwired: 8 in, 1 out]
              n226 = call <vilib>:"Destroy Master Session.vi"("error in (no error)"=w440, "DNP3 master session in"=w453) -> ("error out"=w450:errorcluster)  [unwired: 8 in, 1 out]
              n227 = local write "MS_RESET"(FALSE ("MS_Comm_Reset")) -> ()
              n228 = local write "MS_RESET"(FALSE ("MS_Comm_Reset")) -> ()
              n229 = local write "MS_RESET"(FALSE ("MS_Comm_Reset")) -> ()
              n230 = local write "MS_RESET"(FALSE ("MS_Comm_Reset")) -> ()
              n231 = call <vilib>:"Destroy Master Channel.vi"("error in (no error)"=w450, "DNP3 channel in"=w452) -> ("error out"=w449:errorcluster)  [unwired: 8 in, 1 out]
              n232 = call <vilib>:"Destroy Master.vi"("error in (no error)"=w449, "DNP3 master"=w451) -> ("error out"=w448:errorcluster)  [unwired: 9 in]
              "MS_RESET_IND" <- TRUE ("MS_Comm_Reset_Succesful")
            }
          }
          n233 = Select(t=w405, s=w345, f=w357) -> (s? t:f=w359:errorcluster)
        }
      }
    }
  }
  n234 = local write "Comm Status"(w16) -> ()
  n235 = Bundle("DNP3 channel"=w20, "DNP3 master"=w19, "DNP3 master session"=w18, "DNP3 command"=w15, "MS_Network_Settings_Initial"=w14, "Ping status"=w13, "PollD"=w12, "PollA"=w11, "error out"=w10, "MS_RESET_IND"=w3) -> (w2:T4)  [unwired: 1 in]
  n236 = local write "DNP3 Session Output"(w2) -> ()
